vi "FPGA_DIOWriteDO.vi"(8 "error in (no error)":errorcluster, 10 "DO":u32, 11 "DIODeviceRef":T1) -> (0 "error out":errorcluster, 3 "DIODeviceRef":T1)   [LabVIEW 2017]
uses:
  <vilib>/Rock Robotics/SystemInterfaces/DIO/FPGA_DIODevRef.ctl
  <vilib>/Rock Robotics/SystemInterfaces/System/FPGA_SystemFPGA Ref Global.vi
  <vilib>/Utility/error.llb/Error Cluster From Error Code.vi
  <vilib>/rvi/errors/niLvFpgaAdjustHostInterfaceError.vi
  <vilib>/rvi/interface/nirviReadWriteControl/nirviReadWriteControl.xnode
  <vilib>/Rock Robotics/SystemInterfaces/System/FPGA_SystemFRC FPGA Ref.ctl
  NiFpgaLv.dll
  <vilib>/rvi/interface/Simulation/niFpgaSimulationCallBeginRW.vi
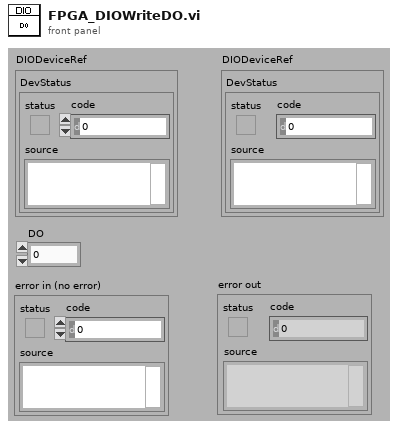
[diagram p1: front panel]
types:
  T1 = typedef "FPGA_DIODevRef.ctl" = cluster{"DevStatus":errorcluster}
  T2 = cluster{"Headers":fxp<+,10,10>, "SPIPort":fxp<+,5,5>, "Reserved":fxp<+,1,1>, "MXP":u16}
  T3 = typedef "FPGA_SystemFRC FPGA Ref.ctl" = refnum<k20>
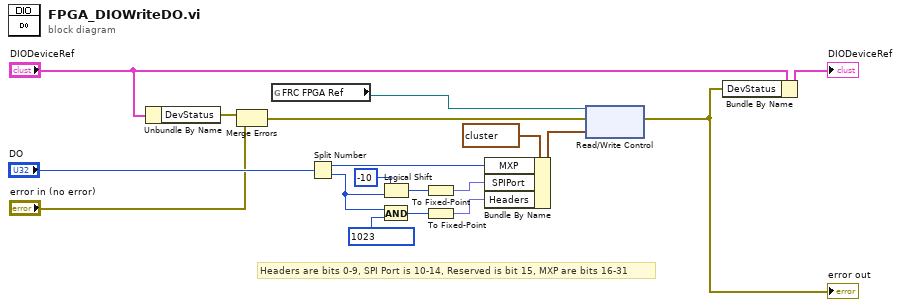
[diagram p0: block diagram]
diagram:
  # "Headers are bits 0-9, SPI Port is 10-14, Reserved is bit 15, MXP are bits 16-31"
  n1 = Unbundle By Name("DIODeviceRef") -> ("DevStatus"=w13:errorcluster)
  n2 = Merge Errors(w13, "error in (no error)") -> (w14:errorcluster)
  n3 = global read "FPGA_SystemFPGA Ref Global.vi" "FRC FPGA Ref"() -> (w15:T3)
  n4 = Split Number(x="DO") -> (hi(x)=w4:u16, lo(x)=w6:u16)
  n5 = Logical Shift(y=i16 -10, x=w6) -> (x << y=w7:u16)
  n6 = And(x=w6, y=u16 1023) -> (x .and. y?=w9:u16)
  n7 = To Fixed-Point(number=w7) -> (fixed-point=w8:fxp<+,5,5>)  [unwired: 1 in]
  n8 = To Fixed-Point(number=w9) -> (fixed-point=w11:fxp<+,10,10>)  [unwired: 1 in]
  n9 = Bundle By Name(cluster=T2 {"Headers"=0.0, "SPIPort"=0.0, "Reserved"=0.0, "MXP"=0} ("DIO.DO"), "MXP"=w4, "SPIPort"=w8, "Headers"=w11) -> (w1:T2)
  n10 = xnode "Read/Write Control"("FPGA VI Reference In"=w15, "error in"=w14, "DIO.DO"=w1) -> ("error out"=w16:errorcluster)  [unwired: 1 out]
  "error out" <- w16
  n11 = Bundle By Name(cluster="DIODeviceRef", "DevStatus"=w16) -> (→"DIODeviceRef":T1)
